vi "ConfigSource.vi"(8 "error in (no error)":errorcluster, 9 "Compliance  Level (0.1)":dbl=0.1, 10 "Voltage Limit (0.0 V)":dbl=1000.0 format="%#_13g", 11 "VISA resource name":refnum<visa-resource-name>) -> (0 "error out":errorcluster, 2 "Output Level (0)":dbl, 3 "VISA resource name out":refnum<visa-resource-name>)   [LabVIEW 2016]
uses:
  instr.lib/Keithley 24XX/Keithley 24XX.lvlib
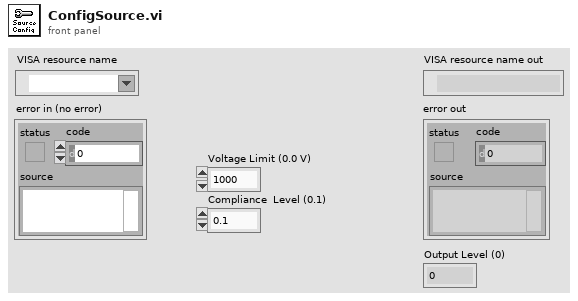
[diagram p1: front panel]
types:
  T1 = cluster{"Baud Rate":u32, "Parity":u16, "Data Bits":u16, "Stop Bits":u16, "Flow Control":u16}
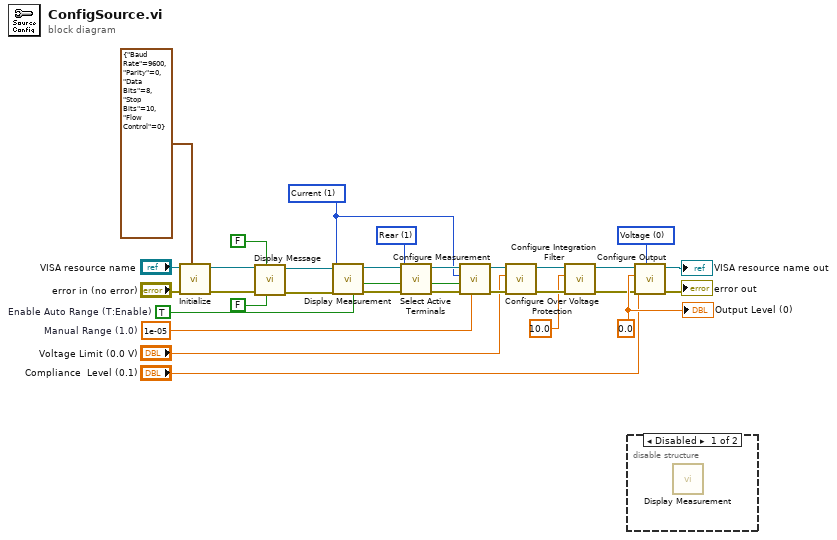
[diagram p0: block diagram]
diagram:
  w8 = 1e-05  # Manual Range (1.0)
  w9 = TRUE  # Enable Auto Range (T:Enable)
  w7 = u16 1 items=["Voltage", "Current", "Resistance"] ("Displayed Measurement (0: Voltage)")
  w17 = u16 1 items=["Front", "Rear"] ("Active Terminals (0: Front)")
  w27 = 0.0 ("Output Level (0)")
  w28 = u16 0 items=["Voltage", "Current"] ("Source Mode  (0: Voltage)")
  n1 = call "Initialize.vi"("Serial Configuration"=T1 {"Baud Rate"=9600, "Parity"=0, "Data Bits"=8, "Stop Bits"=10, "Flow Control"=0}, "error in (no error)"="error in (no error)", "VISA resource name"="VISA resource name") -> ("error out"=w5:errorcluster, "VISA resource name out"=w6:refnum<visa-resource-name>)  [unwired: 7 in]
  n2 = call "Display Message.vi"("Enable Lower Message (T: Enable)"=FALSE, "Enable Upper Message (T: Enable)"=FALSE, "error in (no error)"=w5, "VISA resource name"=w6) -> ("error out"=w4:errorcluster, "VISA resource name out"=w3:refnum<visa-resource-name>)  [unwired: 6 in]
  n3 = call "Display Measurement.vi"("error in (no error)"=w4, "Displayed Measurement (0: Voltage)"=w7, "VISA resource name"=w3) -> ("error out"=w16:errorcluster, "VISA resource name out"=w15:refnum<visa-resource-name>)  [unwired: 7 in]
  n4 = call "Select Active Terminals.vi"("error in (no error)"=w16, "Active Terminals (0: Front)"=w17, "VISA resource name"=w15) -> ("error out"=w18:errorcluster, "VISA resource name out"=w19:refnum<visa-resource-name>)  [unwired: 7 in]
  n5 = call "Configure Measurement.vi"("Manual Range (1.0)"=w8, "error in (no error)"=w18, "Enable Auto Range (T:Enable)"=w9, "Function (0: Volts)"=w7, "VISA resource name"=w19) -> ("error out"=w25:errorcluster, "VISA resource name out"=w26:refnum<visa-resource-name>)  [unwired: 5 in]
  n6 = call "Configure Over Voltage Protection.vi"("error in (no error)"=w25, "Voltage Limit (0.0 V)"="Voltage Limit (0.0 V)", "VISA resource name"=w26) -> ("error out"=w13:errorcluster, "VISA resource name out"=w14:refnum<visa-resource-name>)  [unwired: 7 in]
  n7 = call "Configure Integration Filter.vi"("error in (no error)"=w13, "Measurement Speed (1 PLC)"=10.0, "VISA resource name"=w14) -> ("error out"=w12:errorcluster, "VISA resource name out"=w11:refnum<visa-resource-name>)  [unwired: 7 in]
  n8 = disable-structure shown="Disabled" {
    frame Disabled {
      n9 = call "Display Measurement.vi"() -> ()  [unwired: 10 in, 2 out]
    }
    frame Enabled {
    }
  }
  n10 = call "Configure Output.vi"("Source Mode  (0: Voltage)"=w28, "error in (no error)"=w12, "Compliance  Level (0.1)"="Compliance  Level (0.1)", "Output Level (0)"=w27, "VISA resource name"=w11) -> ("error out"=→"error out":errorcluster, "VISA resource name out"=→"VISA resource name out":refnum<visa-resource-name>)  [unwired: 5 in]
  "Output Level (0)" <- w27
